vi "StyledText.vi"(8 "error in (no error)":errorcluster, 9 "deferPanelUpdates in":bool, 10 "text in":string, 11 "StringControl":refnum<vi>) -> (0 "error out":errorcluster)   [LabVIEW 2010, in "StyledText.lvlib"]
doc: "Writes styled text to the given string control. Supports the following tags to specify styles:\n\n<b ></b > Bold\n<i></i> Italic\n<s></s> or <strike></strike> Strikeout\n<u></u> Underline\n<font></font> Font attributes. Currently supported are face, color and size. Colors must be specified in HTML hexadecimal format.\nExample: <font face=\"Courier\" color=\"#FF0000\" size=\"18\">Blabla</font>\n\n<b>Note that the input text must be well-formed XML content, i.e. every tag must be properly closed and text must be properly escaped.</b>\n\nCopyright (c) 2018, Martin Weiss\nAll rights reserved.\n\nRedistribution and use in source and binary forms, with or without modification, are permitted provided that the following conditions are met:\n\n1. Redistributions of source code must retain the above copyright notice, this list of conditions and the following disclaimer.\n\n2. Redistributions in binary form must reproduce the above copyright notice, this list of conditions and the following disclaimer in the documentation and/or other materials provided with the distribution.\n\nTHIS SOFTWARE IS PROVIDED BY THE COPYRIGHT HOLDERS AND CONTRIBUTORS \"AS IS\" AND ANY EXPRESS OR IMPLIED WARRANTIES, INCLUDING, BUT NOT LIMITED TO, THE IMPLIED WARRANTIES OF MERCHANTABILITY AND FITNESS FOR A PARTICULAR PURPOSE ARE DISCLAIMED. IN NO EVENT SHALL THE COPYRIGHT HOLDER OR CONTRIBUTORS BE LIABLE FOR ANY DIRECT, INDIRECT, INCIDENTAL, SPECIAL, EXEMPLARY, OR CONSEQUENTIAL DAMAGES (INCLUDING, BUT NOT LIMITED TO, PROCUREMENT OF SUBSTITUTE GOODS OR SERVICES; LOSS OF USE, DATA, OR PROFITS; OR BUSINESS INTERRUPTION) HOWEVER CAUSED AND ON ANY THEORY OF LIABILITY, WHETHER IN CONTRACT, STRICT LIABILITY, OR TORT (INCLUDING NEGLIGENCE OR OTHERWISE) ARISING IN ANY WAY OUT OF THE USE OF THIS SOFTWARE, EVEN IF ADVISED OF THE POSSIBILITY OF SUCH DAMAGE."
uses:
  StyledText.lvlib
  TextFragment.ctl
  <vilib>/Utility/miscctls.llb/LVSelectionTypeDef.ctl
  <vilib>/Utility/miscctls.llb/LVFontTypeDef.ctl
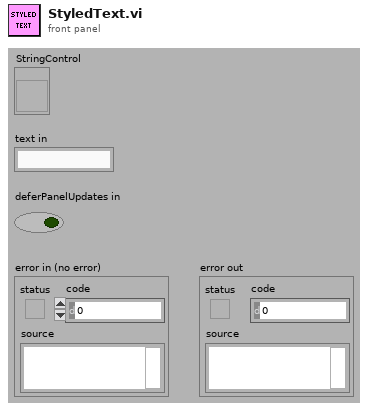
[diagram p1: front panel]
types:
  T1 = typedef "StyledText.lvlib/TextFragment.ctl" = cluster{"text":string, "selection":T2, "font":T3}
  T2 = typedef "LVSelectionTypeDef.ctl" = cluster{"Selection Start":u32, "Selection End":u32}
  T3 = typedef "LVFontTypeDef.ctl" = cluster{"Font Name":string, "Size":u16, "Bold":bool, "Italic":bool, "Underline":bool, "Strikeout":bool, "Color":u32}
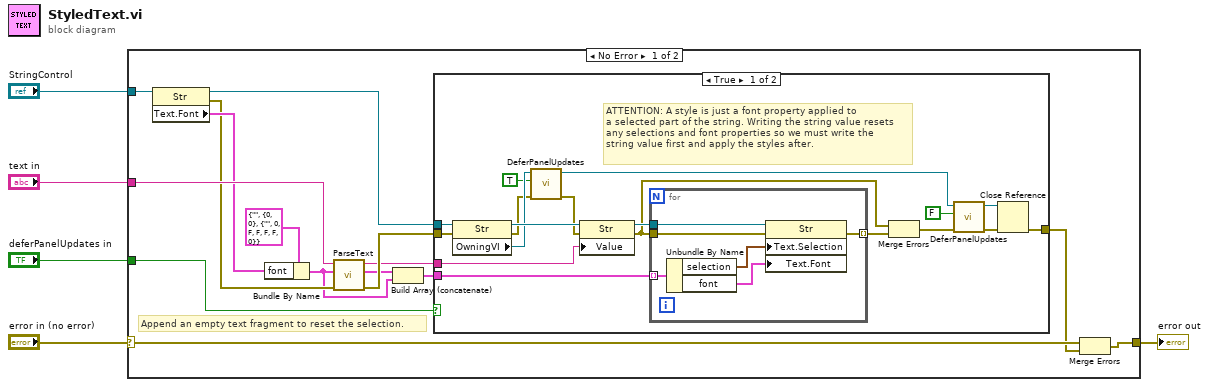
[diagram p0: block diagram]
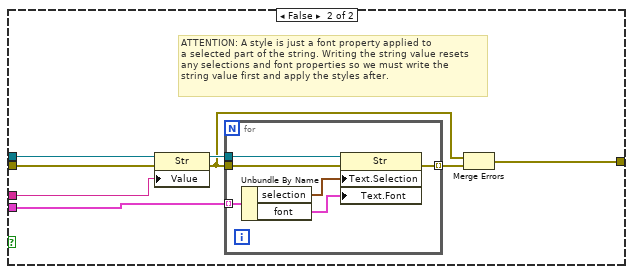
[diagram p2: hidden frame]
diagram:
  n1 = case shown="No Error" "error in (no error)" {
    selector: "error in (no error)" -> [w10 w59]
    tunnel: "text in" -> [w20 _]
    tunnel: [w9 w59] -> w4
    tunnel: "StringControl" -> [w15 _]
    tunnel: "deferPanelUpdates in" -> [w11 _]
    frame No Error {
      # "Append an empty text fragment to reset the selection."
      n2 = property on="Property Node" class="Str"(reference=w15) -> (reference out=w14:refnum<vi>, error out=w16:errorcluster, "Text.Font"=w18:T3)  [unwired: 1 in]
      n3 = Bundle By Name(cluster=T1 {"text"="", "selection"={"Selection Start"=0, "Selection End"=0}, "font"={"Font Name"="", "Size"=0, "Bold"=FALSE, "Italic"=FALSE, "Underline"=FALSE, "Strikeout"=FALSE, "Color"=0}} ("output cluster"), "font"=w18) -> (w6:T1)
      n4 = call "ParseText.vi"("error in (no error)"=w16, "textFragmentDefault in"=w6, "text in"=w20) -> ("error out"=w17:errorcluster, "textFragments out"=w13:T1[], "text out"=w12:string)  [unwired: 6 in]
      n5 = Build Array (concatenate)(w13, w6) -> (w7:T1[])
      n6 = case shown="True" w11 {
        tunnel: w17 -> [w31 w52]
        tunnel: w14 -> [w37 w50]
        tunnel: w7 -> [w36 w49]
        tunnel: w12 -> [w35 w48]
        tunnel: [w30 w45] -> w8
        frame True {
          # "ATTENTION: A style is just a font property applied to\na selected part of the string. Writing the string value resets\nany selections and font properties so we must write the\nstring value first and apply the styles after."
          n7 = property class="Str"(reference=w37, error in=w31) -> (reference out=w32:refnum<vi>, error out=w28:errorcluster, "OwningVI"=w29:refnum<vi>)
          n8 = call "DeferPanelUpdates.vi"("error in"=w28, "deferPanelUpdates in"=TRUE, "VI in"=w29) -> ("error out"=w27:errorcluster, "VI out"=w22:refnum<vi>)  [unwired: 7 in]
          n9 = property on="Property Node" class="Str"(reference=w32, error in=w27, "Value"=w35) -> (reference out=w38:refnum<vi>, error out=w33:errorcluster)
          n10 = for {
            tunnel: w36 -> [w44] mode=indexing
            tunnel: w33 -> [w43]
            tunnel: [w42] -> w34 mode=indexing
            tunnel: w38 -> [w41]
            n11 = Unbundle By Name(w44) -> ("selection"=w40:T2, "font"=w39:T3)
            n12 = property on="Property Node" class="Str"(reference=w41, error in=w43, "Text.Selection"=w40, "Text.Font"=w39) -> (error out=w42:errorcluster)  [unwired: 1 out]
          }
          n13 = Merge Errors(w33, w34) -> (w25:errorcluster)
          n14 = call "DeferPanelUpdates.vi"("error in"=w25, "deferPanelUpdates in"=FALSE, "VI in"=w22) -> ("error out"=w24:errorcluster, "VI out"=w23:refnum<vi>)  [unwired: 7 in]
          n15 = Close Reference(reference=w23, error in (no error)=w24) -> (error out=w30:errorcluster)
        }
        frame False {
          # "ATTENTION: A style is just a font property applied to\na selected part of the string. Writing the string value resets\nany selections and font properties so we must write the\nstring value first and apply the styles after."
          n16 = property on="Property Node" class="Str"(reference=w50, error in=w52, "Value"=w48) -> (reference out=w51:refnum<vi>, error out=w46:errorcluster)
          n17 = for {
            tunnel: w49 -> [w58] mode=indexing
            tunnel: w46 -> [w57]
            tunnel: [w56] -> w47 mode=indexing
            tunnel: w51 -> [w55]
            n18 = Unbundle By Name(w58) -> ("selection"=w54:T2, "font"=w53:T3)
            n19 = property on="Property Node" class="Str"(reference=w55, error in=w57, "Text.Selection"=w54, "Text.Font"=w53) -> (error out=w56:errorcluster)  [unwired: 1 out]
          }
          n20 = Merge Errors(w46, w47) -> (w45:errorcluster)
        }
      }
      n21 = Merge Errors(w10, w8) -> (w9:errorcluster)
    }
    frame Error {
    }
  }
  "error out" <- w4
